vi "CLFNWrapperCloseGateway.vi"(8 "error in (no error)":errorcluster, 10 "ref":i32, 11 "path out":path) -> (0 "error out":errorcluster)   [LabVIEW 2011]
doc: "Execution system set to standard to prevent this DLL from loading in UI thread, which causes labview hang"
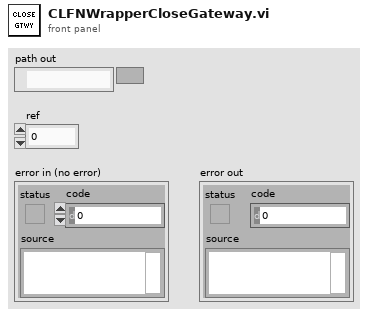
[diagram p1: front panel]
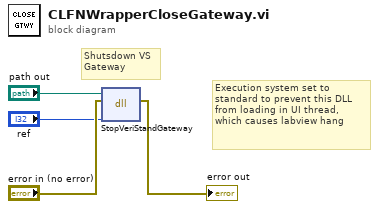
[diagram p0: block diagram]
diagram:
  # "Execution system set to standard to prevent this DLL from loading in UI thread, which causes labview hang"
  # "Shutsdown VS\nGateway"
  n1 = dll-call lib="C:/Program Files (x86)/National Instruments/VeriStand 2010/Data/NationalInstruments.VeriStand.Gateway.dll" fn="StopVeriStandGateway"(path in="path out", error in="error in (no error)", "ref"="ref") -> (error out=→"error out":errorcluster)  [unwired: 3 in, 1 out]
